vi "SET_Example File Format.vi"() -> ()   [LabVIEW 2013]
uses:
  SET Project Data/Types/ProjFile_Project Data.ctl
  SET Project Data/Types/ProjFile_Menu Data.ctl
  SET Project Data/Types/ProjFile_VI Data.ctl
  SET Project Data/Types/ProjFile_GObject Data.ctl
  SET Project Data/Types/ProjFile_Resources Data.ctl
  SET Project Data/Types/ProjFile_Language Entry.ctl
  SET Project Data/Types/ProjFile_Resource Entry.ctl
  SET Project Data/SET Project Data.lvlib
panel:
  out "SET Project File":T8
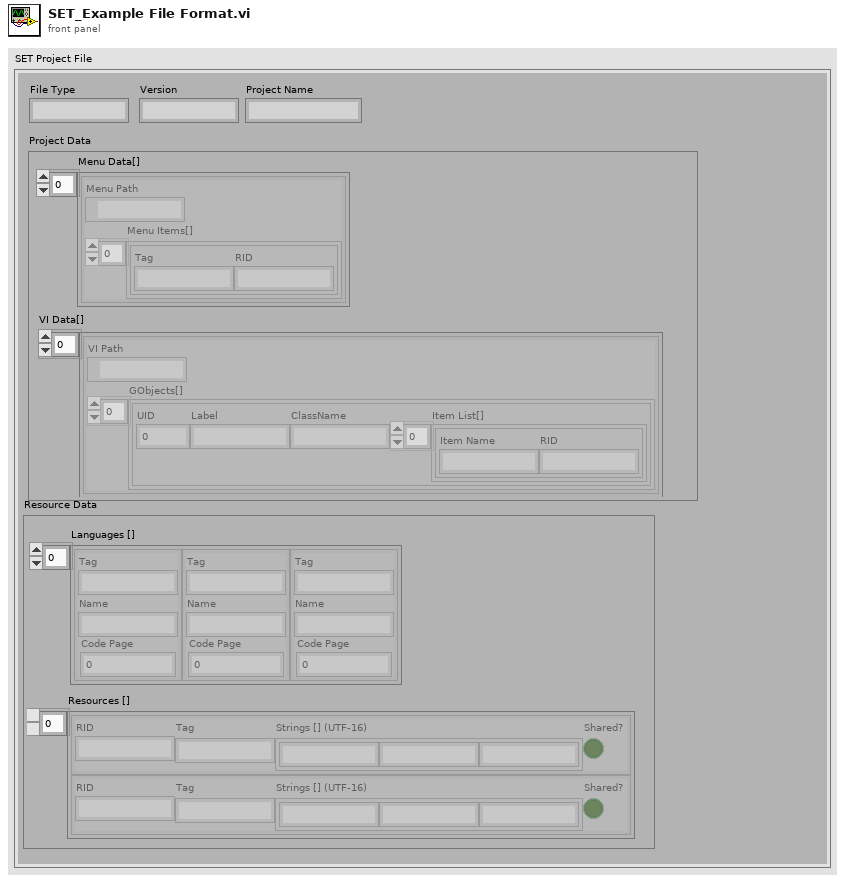
[diagram p1: front panel]
types:
  T1 = typedef "SET Project Data.lvlib/ProjFile_Project Data.ctl" = cluster{"Menu Data[]":T2[], "VI Data[]":T3[]}
  T2 = typedef "SET Project Data.lvlib/ProjFile_Menu Data.ctl" = cluster{"Menu Path":path, "Menu Items[]":cluster{"Tag":string, "RID":string}[]}
  T3 = typedef "SET Project Data.lvlib/ProjFile_VI Data.ctl" = cluster{"VI Path":path, "GObjects[]":T4[]}
  T4 = typedef "SET Project Data.lvlib/ProjFile_GObject Data.ctl" = cluster{"UID":i32, "Label":string, "ClassName":string, "Item List[]":cluster{"Item Name":string, "RID":string}[]}
  T5 = typedef "SET Project Data.lvlib/ProjFile_Resources Data.ctl" = cluster{"Languages []":T6[], "Resources []":T7[]}
  T6 = typedef "SET Project Data.lvlib/ProjFile_Language Entry.ctl" = cluster{"Tag":string, "Name":string, "Code Page":u16}
  T7 = typedef "SET Project Data.lvlib/ProjFile_Resource Entry.ctl" = cluster{"RID":string, "Tag":string, "Strings [] (UTF-16)":string[], "Shared?":bool}
  T8 = cluster{"File Type":string, "Version":string, "Project Name":string, "Project Data":T1, "Resource Data":T5}
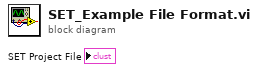
[diagram p0: block diagram]
diagram:
